vi "ERIO RT Process Signal Capture.vi"(6 "Supervisory Variables In":T4={"Alarm Threshold"=0.0, "Shutdown"=FALSE, "Enable SNS Alarm"=FALSE, "Enable SNS Stage Notification"=FALSE, "Enable SQS Notification"=FALSE, "Enable S3 TDMS Signal Capture"=FALSE, "Enable SystemLink Signal Capture"=FALSE, "Capture Signal"=FALSE, "Server Update"=FALSE, "AWS Access Key"="AKIAINLDO2Y2PDFEWDOQ", "AWS Secret Key"="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", "Phone Number"="+15037066913", "Region"=enum."us-west-2", "AWS SQS Queue"="mynicloud-demotest2", "AWS S3 Bucket"="mynicloud-demotest2"}, 7 "RT State":T1, 8 "error in (no error)":errorcluster, 9 "AWS Variables In":T6, 11 "EEISysLink.lvclass In":refnum<class "EEISysLink.lvclass">) -> (0 "error out":errorcluster, 1 "AWS Variables Out":T6, 3 "EEISysLink.lvclass Out":refnum<class "EEISysLink.lvclass">, 4 "Supervisory Variables Out":T4={"Alarm Threshold"=0.0, "Shutdown"=FALSE, "Enable SNS Alarm"=FALSE, "Enable SNS Stage Notification"=FALSE, "Enable SQS Notification"=FALSE, "Enable S3 TDMS Signal Capture"=FALSE, "Enable SystemLink Signal Capture"=FALSE, "Capture Signal"=FALSE, "Server Update"=FALSE, "AWS Access Key"="AKIAINLDO2Y2PDFEWDOQ", "AWS Secret Key"="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", "Phone Number"="+15037066913", "Region"=enum."us-west-2", "AWS SQS Queue"="mynicloud-demotest2", "AWS S3 Bucket"="mynicloud-demotest2"}, 5 "Last Triggered Signal Capture":waveform(dbl))   [LabVIEW 2017]
doc: "Process the last signal update for potential signal capture snapshot to be distributed as enabled. \n\nJames Tillett P.E.\nEndeavor Engineering Inc.\nwww.endeavoreng.com"
uses:
  Class EEISysLink/EEISysLink.lvclass
  Controls/ERIO AWS Toolkit Variables.ctl
  <vilib>/AWS Toolkit/SQS/Queue/Queue.lvclass
  <vilib>/AWS Toolkit/SNS/Phone Number/Phone Number.lvclass
  <vilib>/AWS Toolkit/S3/Bucket/Bucket.lvclass
  Controls/ERIO Supervisory Variables.ctl
  <vilib>/AWS Toolkit/Core/HTTP Request/Region.ctl
  Controls/ERIO RT State Variables.ctl
  Controls/ERIO SystemStates.ctl
  Controls/ERIO Queue Data.ctl
  Controls/ERIO Worker Variables.ctl
  Class EEISysLink/Controls/SL Tag Type.ctl
  Class EEISysLink/Controls/SL Tag Scope.ctl
  <vilib>/AWS Toolkit/Core/HTTP Request/HTTP Request.lvclass
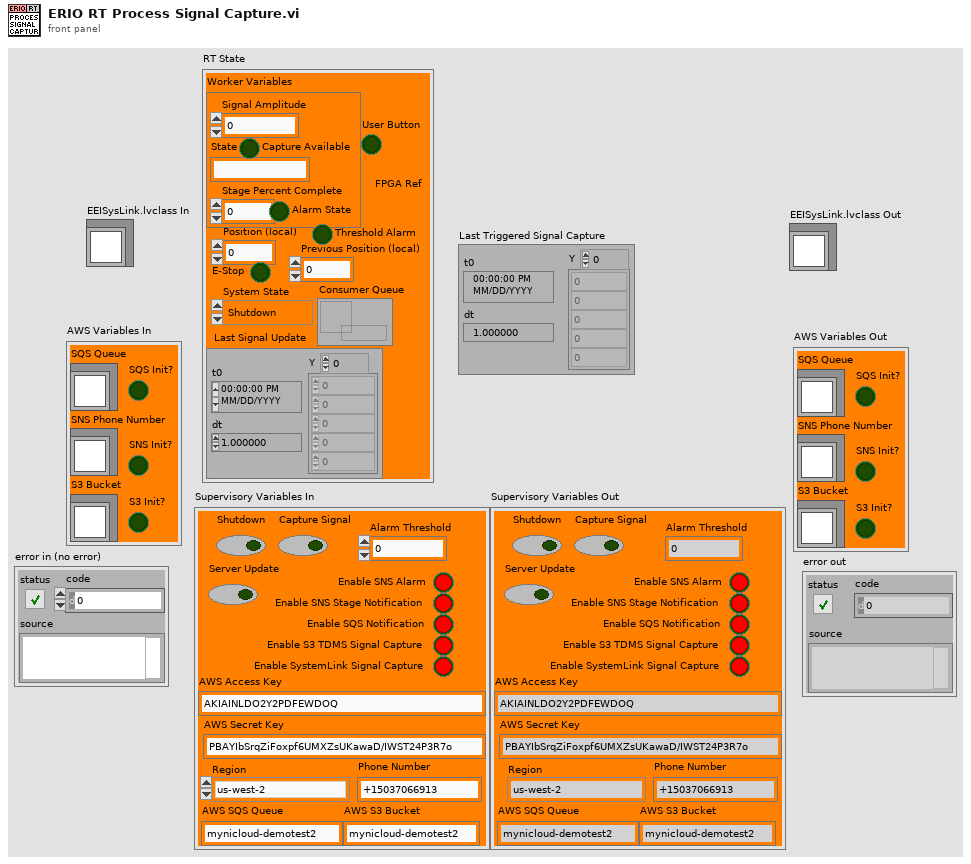
[diagram p1: front panel]
types:
  T1 = typedef "ERIO RT State Variables.ctl" = cluster{"Position (local)":i16, "E-Stop":bool, "System State":T2, "FPGA Ref":refnum<k20>, "Previous Position (local)":i16, "Consumer Queue":refnum<queue>, "Worker Variables":T3, "Threshold Alarm":bool, "User Button":bool, "Last Signal Update":waveform(dbl)}
  T2 = typedef "ERIO SystemStates.ctl" = enum16{"Shutdown", "E-STOP", "Reset Process", "Stage 1", "Stage 2", "Stage 3", "Alarm State"}
  T3 = typedef "ERIO Worker Variables.ctl" = cluster{"Signal Amplitude":dbl, "State":string, "Stage Percent Complete":dbl, "Alarm State":bool, "Capture Available":bool}
  T4 = typedef "ERIO Supervisory Variables.ctl" = cluster{"Alarm Threshold":dbl, "Shutdown":bool, "Enable SNS Alarm":bool, "Enable SNS Stage Notification":bool, "Enable SQS Notification":bool, "Enable S3 TDMS Signal Capture":bool, "Enable SystemLink Signal Capture":bool, "Capture Signal":bool, "Server Update":bool, "AWS Access Key":string, "AWS Secret Key":string, "Phone Number":string, "Region":T5, "AWS SQS Queue":string, "AWS S3 Bucket":string}
  T5 = typedef "NI_AWS_Core.lvlib/HTTP Request.lvclass/Region.ctl" = enum16{"us-east-1", "us-east-2", "us-west-1", "us-west-2", "ap-northeast-1", "ap-northeast-2", "ap-southeast-1", "ap-southeast-2", "ca-central-1", "eu-central-1", "eu-west-1", "eu-west-2", "sa-east-1"}
  T6 = typedef "ERIO AWS Toolkit Variables.ctl" = cluster{"SQS Queue":refnum<class "Queue.lvclass">, "SNS Phone Number":refnum<class "Phone Number.lvclass">, "S3 Bucket":refnum<class "Bucket.lvclass">, "SQS Init?":bool, "S3 Init?":bool, "SNS Init?":bool}
  T7 = typedef "EEISysLink.lvclass/SL Tag Scope.ctl" = enum16{"Local", "Server"}
  T8 = typedef "EEISysLink.lvclass/SL Tag Type.ctl" = enum16{"All", "Supervisor", "Worker"}
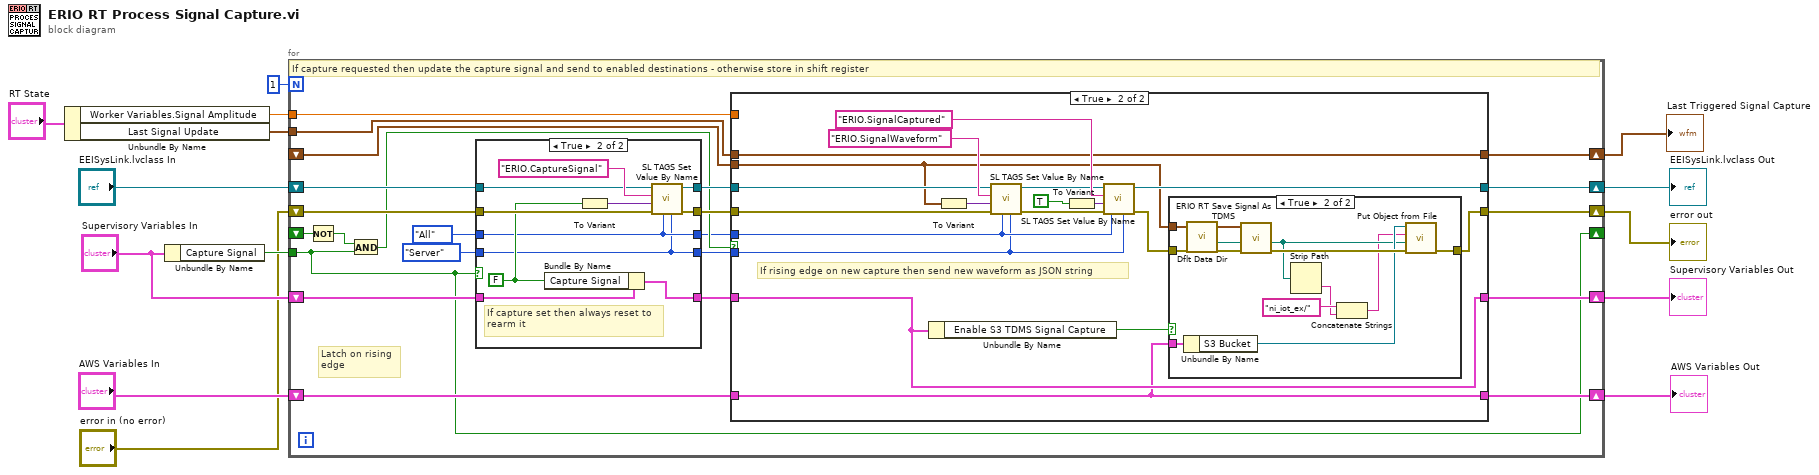
[diagram p0: block diagram]
diagram:
  n1 = Unbundle By Name("RT State") -> ("Worker Variables.Signal Amplitude"=w3:dbl, "Last Signal Update"=w2:waveform(dbl))
  n2 = Unbundle By Name("Supervisory Variables In") -> ("Capture Signal"=w14:bool)
  n3 = for {
    N: 1 -> [_]
    tunnel: w14 -> [w19]
    tunnel: w3 -> [w37]
    shift-right: [w36] -> w5
    shift-left: _ -> [w27]
    shift-right: [w34] -> w10
    shift-left: "EEISysLink.lvclass In" -> [w26]
    shift-right: [w35] -> w9
    shift-left: "error in (no error)" -> [w25]
    shift-right: [w33] -> w8
    shift-left: "Supervisory Variables In" -> [w24]
    shift-right: [w31] -> w6
    shift-left: "AWS Variables In" -> [w32]
    tunnel: w2 -> [w28]
    shift-right: [w19] -> _
    shift-left: _ -> [w30]
    # "Latch on rising\nedge"
    # "If capture requested then update the capture signal and send to enabled destinations - otherwise store in shift register"
    n4 = Not(x=w30) -> (.not. x?=w29:bool)
    n5 = And(x=w29, y=w19) -> (x .and. y?=w20:bool)
    n6 = case shown="True" w19 {
      tunnel: w24 -> [w40 w49]
      tunnel: w26 -> [w42 w51]
      tunnel: w25 -> [w41 w50]
      tunnel: [w41 w45] -> w22
      tunnel: [w42 w46] -> w23
      tunnel: [w40 w48] -> w21
      tunnel: SL_Tag_Type."All" ("Tag Type") -> [w39 w44]
      tunnel: SL_Tag_Scope."Server" ("Tag Scope") -> [w38 w43]
      tunnel: [w39 w44] -> w16
      tunnel: [w38 w43] -> w15
      frame False {
        # "No capture requested so just \nreturn same values"
      }
      frame True {
        w47 = FALSE ("Capture Signal")
        # "If capture set then always reset to\nrearm it"
        n7 = Bundle By Name(cluster=w49, "Capture Signal"=w47) -> (w48:T4)
        n8 = To Variant(anything=w47) -> (Variant=w52:variant)
        n9 = call-dynamic "SL TAGS Set Value By Name.vi"("Tag Scope"=w43, "Tag Type"=w44, "error in (no error)"=w50, "Value"=w52, "Tag Name"="ERIO.CaptureSignal", "EEISysLink in"=w51) -> ("error out"=w45:errorcluster, "EEISysLink out"=w46:refnum<class "EEISysLink.lvclass">)  [unwired: 4 in]
      }
    }
    n10 = case shown="True" w20 {
      tunnel: w37 -> [_ _]
      tunnel: w27 -> [w58 w61]
      tunnel: [w58 w70] -> w36
      tunnel: w21 -> [w55 w64]
      tunnel: w23 -> [w57 w66]
      tunnel: w22 -> [w56 w65]
      tunnel: [w56 w59] -> w35
      tunnel: [w57 w75] -> w34
      tunnel: [w55 w64] -> w33
      tunnel: [w54 w62] -> w31
      tunnel: w32 -> [w54 w62]
      tunnel: w28 -> [_ w70]
      tunnel: w16 -> [_ w68]
      tunnel: w15 -> [_ w67]
      frame False {
        # "No capture requested so just return same values"
      }
      frame True {
        # "If rising edge on new capture then send new waveform as JSON string"
        n11 = Unbundle By Name(w64) -> ("Enable S3 TDMS Signal Capture"=w63:bool)
        n12 = To Variant(anything=w61) -> (Variant=w74:variant)
        n13 = call-dynamic "SL TAGS Set Value By Name.vi"("Tag Scope"=w67, "Tag Type"=w68, "error in (no error)"=w65, "Value"=w74, "Tag Name"="ERIO.SignalWaveform", "EEISysLink in"=w66) -> ("error out"=w72:errorcluster, "EEISysLink out"=w71:refnum<class "EEISysLink.lvclass">)  [unwired: 4 in]
        n14 = To Variant(anything=TRUE ("Capture Signal")) -> (Variant=w76:variant)
        n15 = call-dynamic "SL TAGS Set Value By Name.vi"("Tag Scope"=w67, "Tag Type"=w68, "error in (no error)"=w72, "Value"=w76, "Tag Name"="ERIO.SignalCaptured", "EEISysLink in"=w71) -> ("error out"=w60:errorcluster, "EEISysLink out"=w75:refnum<class "EEISysLink.lvclass">)  [unwired: 4 in]
        n16 = case shown="True" w63 {
          tunnel: w62 -> [_ w89]
          tunnel: w61 -> [_ w88]
          tunnel: w60 -> [w78 w87]
          tunnel: [w78 w79] -> w59
          frame False {
          }
          frame True {
            n17 = Unbundle By Name(w89) -> ("S3 Bucket"=w84:refnum<class "Bucket.lvclass">)
            n18 = call <vilib>:"Dflt Data Dir.vi"() -> ("App:Default Data Directory"=w86:path)
            n19 = call "ERIO RT Save Signal As TDMS.vi"("error in (no error)"=w87, "TDMS File Folder In"=w86, "Signal Capture"=w88) -> ("error out"=w85:errorcluster, "TDMS File Path Out"=w83:path)  [unwired: 7 in]
            n20 = Strip Path(path=w83) -> (name=w81:string)  [unwired: 1 out]
            n21 = Concatenate Strings("ni_iot_ex/", w81) -> (w80:string)
            n22 = call <vilib>:"Put Object from File.vi"("error in (no error)"=w85, "File"=w83, "Object Path"=w80, "Bucket in"=w84) -> ("error out"=w79:errorcluster)  [unwired: 3 in, 4 out]
          }
        }
      }
    }
  }
  "EEISysLink.lvclass Out" <- w10
  "error out" <- w9
  "AWS Variables Out" <- w6
  "Supervisory Variables Out" <- w8
  "Last Triggered Signal Capture" <- w5
